vi "CANOpen_State_Opp_Preopp.vi"(11 "state":u16(ring) items=["unknown"=1, "bootup"=0, "stopped"=4, "operational"=5, "pre-operational"=127, "connection lost"=128]) -> (3 "Active":bool)   [LabVIEW 2013, in "CANOpen Addon Custom Device.lvlib"]
uses:
  CANOpen Addon Custom Device.lvlib
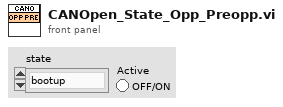
[diagram p1: front panel]
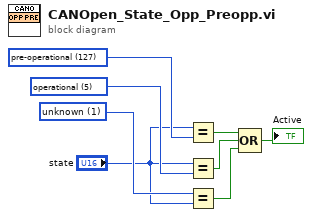
[diagram p0: block diagram]
diagram:
  w3 = u16 1 items=["unknown"=1, "bootup"=0, "stopped"=4, "operational"=5, "pre-operational"=127, "connection lost"=128] ("state")
  w4 = u16 5 items=["unknown"=1, "bootup"=0, "stopped"=4, "operational"=5, "pre-operational"=127, "connection lost"=128] ("state")
  w5 = u16 127 items=["unknown"=1, "bootup"=0, "stopped"=4, "operational"=5, "pre-operational"=127, "connection lost"=128] ("state")
  n1 = Equal?(x="state", y=w5) -> (x = y?=w7:bool)
  n2 = Equal?(x="state", y=w4) -> (x = y?=w8:bool)
  n3 = Equal?(x=w3, y="state") -> (x = y?=w1:bool)
  n4 = Compound Arithmetic op=OR(w7, w8, w1) -> (→"Active":bool)
